vi "DMA.Scatter-Gather.Link Block Descriptors.vi"(8 "error in (no error)":errorcluster, 10 "Block Descriptors":T1[](array[typedef]) {"next descriptor ptr" format="%08x"; "data size" format="%08x"; "data ptr (upper)" format="%08x"; "data ptr (lower)" format="%08x"; "descriptor ptr (aligned)" format="%08x"; "descriptor size" format="%08x"; "descriptor ptr (VISA)" format="%08x"}, 11 "GE 5565PIORC in":refnum<class "GE 5565PIORC.lvclass">) -> (0 "error out":errorcluster, 2 "Block Descriptors out":T1[](array[typedef]) {"next descriptor ptr" format="%08x"; "data size" format="%08x"; "data ptr (upper)" format="%08x"; "data ptr (lower)" format="%08x"; "descriptor ptr (aligned)" format="%08x"; "descriptor size" format="%08x"; "descriptor ptr (VISA)" format="%08x"}, 3 "GE 5565PIORC out":refnum<class "GE 5565PIORC.lvclass">)   [LabVIEW 2016, in "GE 5565PIORC.lvclass"]
uses:
  GE 5565PIORC.lvclass
  Controls/DMA Block Descriptor.ctl
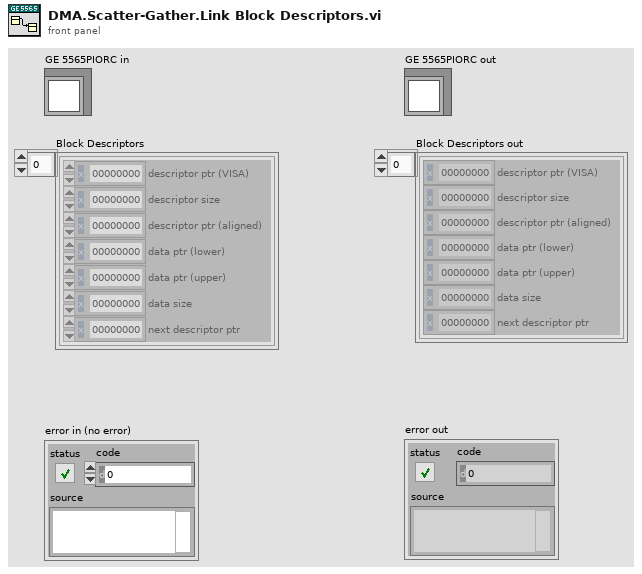
[diagram p1: front panel]
types:
  T1 = typedef "GE 5565PIORC.lvclass/DMA Block Descriptor.ctl" = cluster{"descriptor ptr (VISA)":u32, "descriptor size":u32, "descriptor ptr (aligned)":u32, "data ptr (lower)":u32, "data ptr (upper)":u32, "data size":u32, "next descriptor ptr":u32}
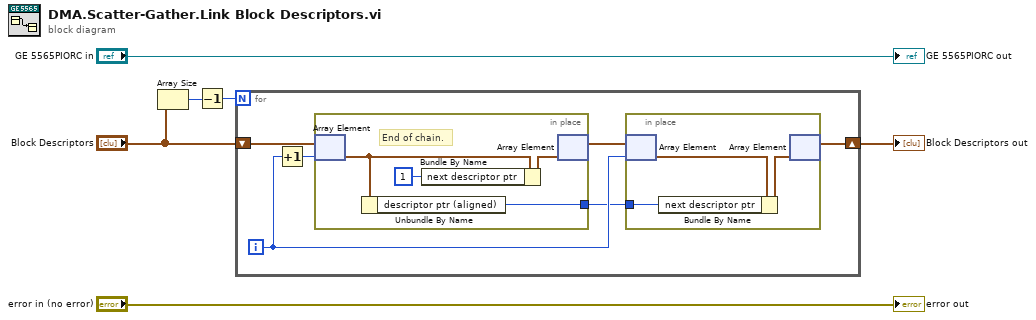
[diagram p0: block diagram]
diagram:
  n1 = Array Size(array="Block Descriptors") -> (size(s)=w4:i32)
  n2 = Decrement(x=w4) -> (x-1=w3:i32)
  n3 = for {
    N: w3 -> [_]
    shift-right: [w8] -> w2
    shift-left: "Block Descriptors" -> [w11]
    i -> [w9]
    n4 = Increment(x=w9) -> (x+1=w12:i32)
    n5 = in-place {
      in-place-border: [w16] -> w7
      # "End of chain."
      n6 = in-place-array #1(w11, w12) -> (w19:T1)
      n7 = Unbundle By Name(w19) -> ("descriptor ptr (aligned)"=w16:u32)
      n8 = Bundle By Name(cluster=w19, "next descriptor ptr"=u32 1) -> (w18:T1)
      n9 = in-place-array #1(w18) -> (w10:T1[])  [unwired: 1 out]
    }
    n10 = in-place {
      in-place-border: w7 -> [w13]
      n11 = in-place-array #2(w10, w9) -> (w15:T1)
      n12 = Bundle By Name(cluster=w15, "next descriptor ptr"=w13) -> (w14:T1)
      n13 = in-place-array #2(w14) -> (w8:T1[])  [unwired: 1 out]
    }
  }
  "Block Descriptors out" <- w2
  "error out" <- "error in (no error)"
  "GE 5565PIORC out" <- "GE 5565PIORC in"
